vi "Create_Object.vi"(8 "error in (no error)":errorcluster, 9 "Block Diagram in":T1, 10 "owner refnum":variant, 11 "Loop in":refnum<class "Loop.lvclass">) -> (0 "error out":errorcluster, 1 "Block Diagram Out":T1, 3 "Loop out":refnum<class "Loop.lvclass">)   [LabVIEW 2025, in "Loop.lvclass"]
uses:
  Loop.lvclass
  Controls/bd.ctl
  Node.lvclass
  Controls/wire.ctl
  Controls/Terminal.ctl
  Structure.lvclass
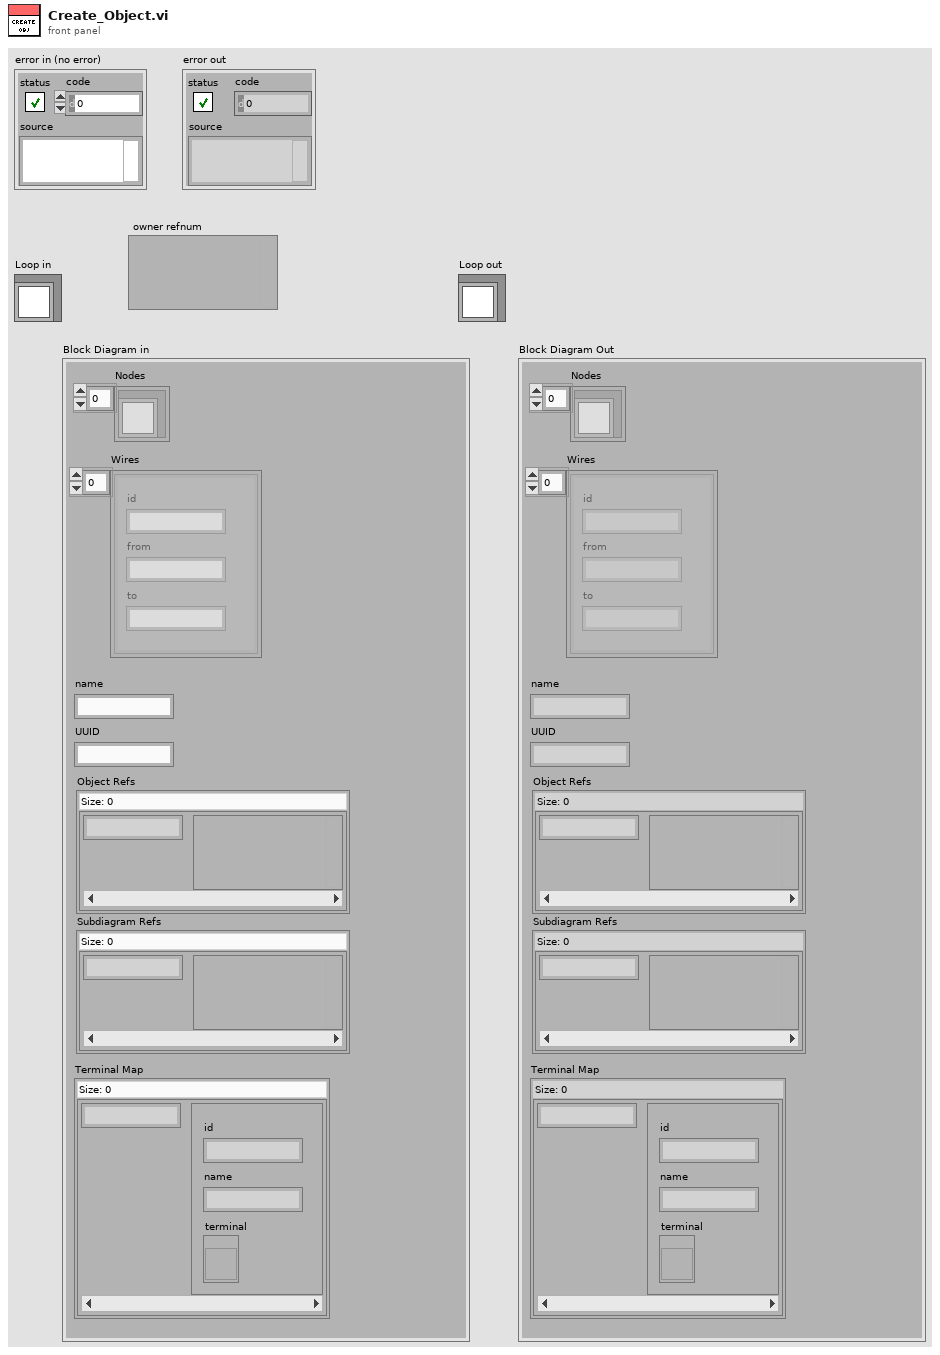
[diagram p1: front panel]
types:
  T1 = typedef "bd.ctl" = cluster{"Nodes":refnum<class "Node.lvclass">[], "Wires":T2[], "name":string, "UUID":string, "Object Refs":map{string, variant}, "Subdiagram Refs":map{string, variant}, "Terminal Map":map{string, T3}}
  T2 = typedef "wire.ctl" = cluster{"id":string, "from":string, "to":string}
  T3 = typedef "Terminal.ctl" = cluster{"id":string, "name":string, "terminal":refnum<vi>}
  T4 = typedef "Shift Register.ctl" = cluster{"name":string, "LH Ext":T3, "LH Int":T3, "RH Int":T3, "RH Ext":T3, "Y pos":u32}
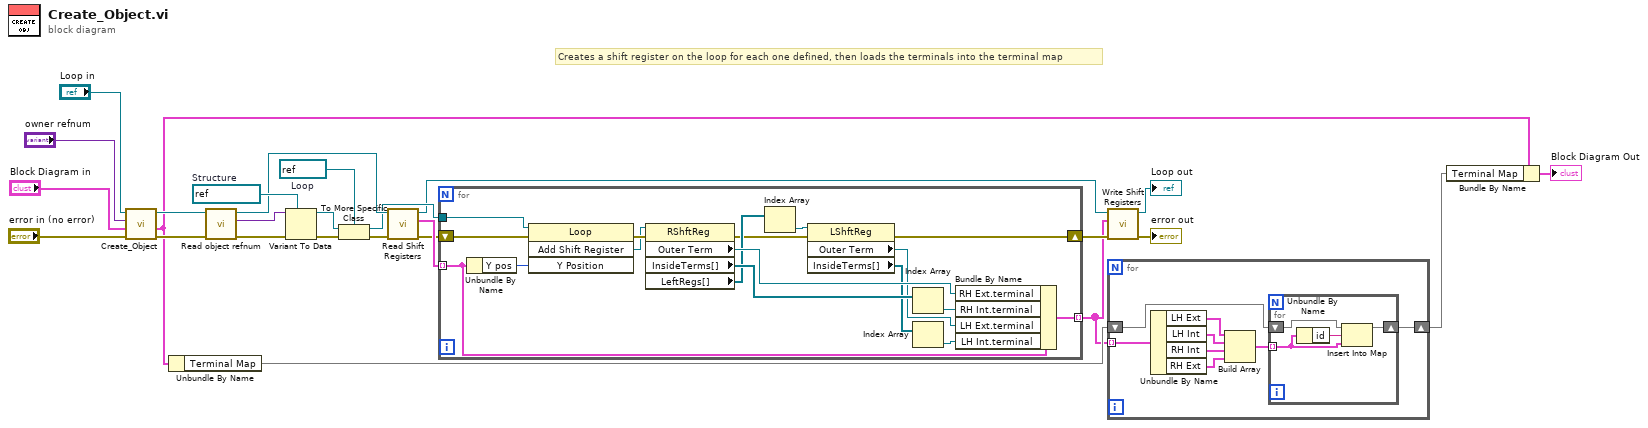
[diagram p0: block diagram]
diagram:
  w15 = refnum<vi> refnum  # Loop
  w18 = refnum<vi> refnum  # Structure
  # "Creates a shift register on the loop for each one defined, then loads the terminals into the terminal map"
  n1 = call-parent "Create_Object.vi"("error in (no error)"="error in (no error)", "Block Diagram in"="Block Diagram in", "owner refnum"="owner refnum", "Structure in"="Loop in") -> ("error out"=w22:errorcluster, "Block Diagram Out"=w4:T1, "Structure out"=w21:refnum<class "Loop.lvclass">)  [unwired: 5 in]
  n2 = Unbundle By Name(w4) -> ("Terminal Map"=w7:map{string, T3})
  n3 = call-dynamic "Read object refnum.vi"("error in (no error)"=w22, "Node in"=w21) -> ("error out"=w19:errorcluster, "object refnum"=w20:variant, "Node out"=w14:refnum<class "Loop.lvclass">)  [unwired: 7 in]
  n4 = Variant To Data(error in=w19, type=w18, Variant=w20) -> (data=w16:refnum<vi>, error out=w17:errorcluster)
  n5 = To More Specific Class(target class=w15, reference=w16, error in=w17) -> (specific class reference=w11:refnum<vi>, error out=w13:errorcluster)
  n6 = call-dynamic "Read Shift Registers.vi"("error in (no error)"=w13, "Loop in"=w14) -> ("error out"=w10:errorcluster, "Shift Registers"=w12:T4[], "Loop out"=w8:refnum<class "Loop.lvclass">)  [unwired: 7 in]
  n7 = for {
    tunnel: w12 -> [w38] mode=indexing
    tunnel: w11 -> [w43]
    shift-right: [w28] -> w9
    shift-left: w10 -> [w41]
    tunnel: [w27] -> w5 mode=indexing
    n8 = Unbundle By Name(w38) -> ("Y pos"=w42:u32)
    n9 = invoke class="Loop" method="Add Shift Register"(reference=w43, error in=w41, "Y Position"=w42) -> (error out=w40:errorcluster, "Add Shift Register"=w39:refnum<vi>)  [unwired: 1 in, 2 out]
    n10 = property class="RShftReg"(reference=w39, error in=w40) -> (error out=w33:errorcluster, "Outer Term"=w36:refnum<vi>, "InsideTerms[]"=w37:refnum<vi>[], "LeftRegs[]"=w34:refnum<vi>[])  [unwired: 1 out]
    n11 = Index Array(array=w34) -> (element=w32:refnum<vi>)  [unwired: 1 in]
    n12 = property class="LShftReg"(reference=w32, error in=w33) -> (error out=w28:errorcluster, "Outer Term"=w30:refnum<vi>, "InsideTerms[]"=w31:refnum<vi>[])  [unwired: 1 out]
    n13 = Index Array(array=w37) -> (element=w35:refnum<vi>)  [unwired: 1 in]
    n14 = Index Array(array=w31) -> (element=w29:refnum<vi>)  [unwired: 1 in]
    n15 = Bundle By Name(cluster=w38, "RH Ext.terminal"=w36, "RH Int.terminal"=w35, "LH Ext.terminal"=w30, "LH Int.terminal"=w29) -> (w27:T4)
  }
  n16 = call-dynamic "Write Shift Registers.vi"("error in (no error)"=w9, "Shift Registers"=w5, "Loop in"=w8) -> ("error out"=→"error out":errorcluster, "Loop out"=→"Loop out":refnum<class "Loop.lvclass">)  [unwired: 7 in]
  n17 = for {
    shift-right: [w44] -> w3
    shift-left: w7 -> [w45]
    tunnel: w5 -> [w51] mode=indexing
    n18 = Unbundle By Name(w51) -> ("LH Ext"=w50:T3, "LH Int"=w49:T3, "RH Int"=w48:T3, "RH Ext"=w47:T3)
    n19 = Build Array(w50, w49, w48, w47) -> (w46:T3[])
    n20 = for {
      tunnel: w46 -> [w52] mode=indexing
      shift-right: [w54] -> w44
      shift-left: w45 -> [w55]
      n21 = Unbundle By Name(w52) -> ("id"=w53:string)
      n22 = Insert Into Map(map in=w55, key=w53, value=w52) -> (map out=w54:map{string, T3})  [unwired: 2 out]
    }
  }
  n23 = Bundle By Name(cluster=w4, "Terminal Map"=w3) -> (→"Block Diagram Out":T1)
